vi "Solutions FM Demodulation.vi"(8 "错误输入":errorcluster, 10 "重采样率":dbl, 11 "接收信号":waveform(cdb)) -> (0 "错误输出":errorcluster, 2 "重采样后信号":waveform(dbl)(graph), 3 "解调后信号":waveform(dbl)(graph))   [LabVIEW 2015]
uses:
  <vilib>/measure/maresamp.llb/Resample Waveform (continuous).vi
  <vilib>/measure/NI_MAPro.lvlib
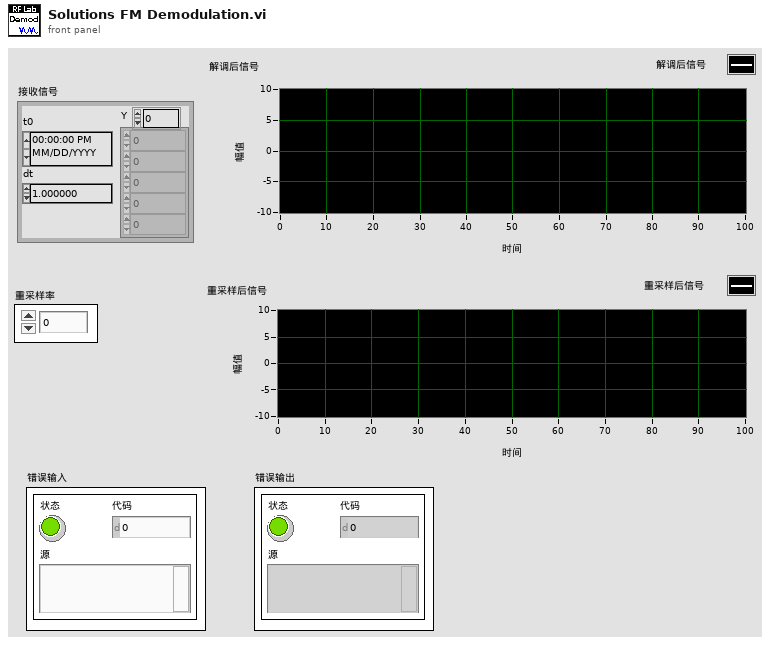
[diagram p1: front panel]
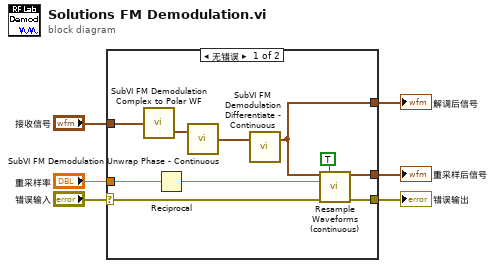
[diagram p0: block diagram]
diagram:
  n1 = case shown="无错误" "错误输入" {
    selector: "错误输入" -> [w7 w17]
    tunnel: "接收信号" -> [w16 _]
    tunnel: "重采样率" -> [w14 _]
    tunnel: [w12 _] -> w4
    tunnel: [w10 _] -> w3
    tunnel: [w9 w17] -> w2
    frame No Error {
      n2 = call "SubVI FM Demodulation Complex to Polar WF.vi"("输入信号"=w16) -> ("相角"=w13:waveform(dbl))  [unwired: 1 out]
      n3 = Reciprocal(x=w14) -> (1/x=w11:dbl)
      n4 = call "SubVI FM Demodulation Unwrap Phase - Continuous.vi"("输入信号"=w13) -> ("相位展开"=w15:waveform(dbl))  [unwired: 1 in]
      n5 = call "SubVI FM Demodulation Differentiate - Continuous.vi"("输入信号"=w15) -> ("dx/dt"=w12:waveform(dbl))  [unwired: 2 in]
      n6 = call-poly <vilib>:"Resample Waveforms (continuous).vi"("waveform in"=w12, "reset"=TRUE, "dt"=w11, "error in (no error)"=w7) -> ("resampled waveform out"=w10:waveform(dbl), "error out"=w9:errorcluster)  [unwired: 7 in, 3 out]
    }
    frame Error {
    }
  }
  "重采样后信号" <- w3
  "解调后信号" <- w4
  "错误输出" <- w2
